vi "CMC_Homework_02.vi"() -> ()   [LabVIEW 2013]
doc: "Simulates the hardware controls for a manufacturing machine\nCreated in part with the collaboration of Sarah Bailey & Alex Offredi"
panel:
  in  "Max Tank Pressure":dbl(knob)=875.0 scale=0.0..10.0
  in  "Max Tank Temp":dbl(knob)=550.0 scale=0.0..10.0
  in  "Max Ps":dbl(knob)=700.0 scale=0.0..10.0
  in  "Max Ts":dbl(knob)=230.0 scale=0.0..10.0
  in  "Tank Pressure":dbl(knob) step=1.0 scale=0.0..1000.0
  in  "Tank Temp":dbl(knob) step=1.0 scale=0.0..1000.0
  out "Status":string
  in  "stop":bool
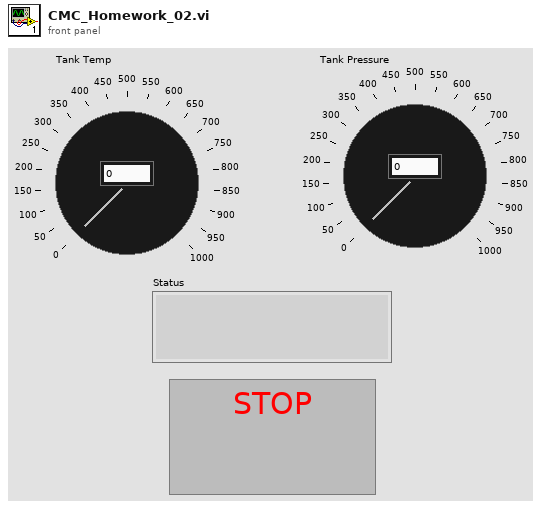
[diagram p1: front panel]
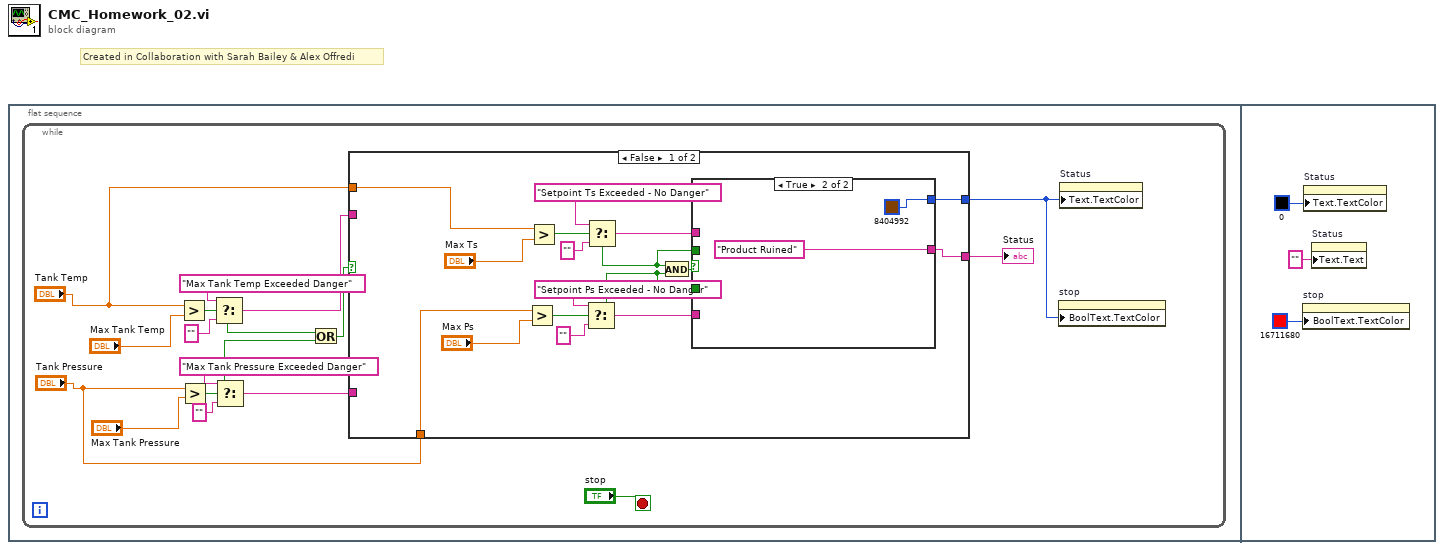
[diagram p0: block diagram]
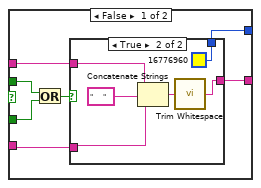
[diagram p2: hidden frame]
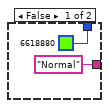
[diagram p3: hidden frame]
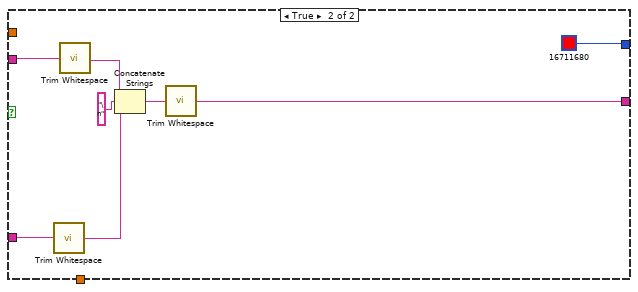
[diagram p4: hidden frame]
diagram:
  # "Created in Collaboration with Sarah Bailey & Alex Offredi"
  n1 = flat-sequence {
    frame #0 {
      n2 = while {
        stop <- "stop" stop-if-true
        n3 = Greater?(x="Tank Temp", y="Max Tank Temp") -> (0:w10:bool)
        n4 = Greater?(x="Tank Pressure", y="Max Tank Pressure") -> (0:w9:bool)
        n5 = Select(t="Max Tank Temp Exceeded Danger", s=w10, f="") -> (s? t:f=w7:string)
        n6 = Select(t="Max Tank Pressure Exceeded Danger", s=w9, f="") -> (s? t:f=w6:string)
        n7 = Or(x=w10, y=w9) -> (x .or. y?=w8:bool)
        n8 = case shown="False" w8 {
          tunnel: w7 -> [_ w53]
          tunnel: w6 -> [_ w52]
          tunnel: [w20 w49] -> w5
          tunnel: "Tank Temp" -> [w19 _]
          tunnel: "Tank Pressure" -> [w18 _]
          tunnel: [w17 u32 16711680] -> w1
          frame False {
            n9 = Greater?(x=w18, y="Max Ps") -> (0:w21:bool)
            n10 = Greater?(x=w19, y="Max Ts") -> (0:w22:bool)
            n11 = Select(t="Setpoint Ps Exceeded - No Danger", s=w21, f="") -> (s? t:f=w23:string)
            n12 = Select(t="Setpoint Ts Exceeded - No Danger", s=w22, f="") -> (s? t:f=w24:string)
            n13 = And(x=w22, y=w21) -> (x .and. y?=w25:bool)
            n14 = case shown="True" w25 {
              tunnel: w24 -> [w35 _]
              tunnel: w23 -> [w34 _]
              tunnel: [w33 "Product Ruined"] -> w20
              tunnel: w22 -> [w37 _]
              tunnel: w21 -> [w36 _]
              tunnel: [w32 u32 8404992] -> w17
              frame False {
                n15 = Or(x=w37, y=w36) -> (x .or. y?=w38:bool)
                n16 = case shown="True" w38 {
                  tunnel: w35 -> [_ w46]
                  tunnel: w34 -> [_ w45]
                  tunnel: ["Normal" w42] -> w33
                  tunnel: [u32 6618880 u32 16776960] -> w32
                  frame False {
                  }
                  frame True {
                    n17 = Concatenate Strings(w46, "     ", w45) -> (w43:string)
                    n18 = call <vilib>:"Trim Whitespace.vi"("string"=w43) -> ("trimmed string"=w42:string)  [unwired: 1 in]
                  }
                }
              }
              frame True {
              }
            }
          }
          frame True {
            n19 = call <vilib>:"Trim Whitespace.vi"("string"=w52) -> ("trimmed string"=w51:string)  [unwired: 1 in]
            n20 = call <vilib>:"Trim Whitespace.vi"("string"=w53) -> ("trimmed string"=w54:string)  [unwired: 1 in]
            n21 = Concatenate Strings(w54, "\n" ("string"), w51) -> (w50:string)
            n22 = call <vilib>:"Trim Whitespace.vi"("string"=w50) -> ("trimmed string"=w49:string)  [unwired: 1 in]
          }
        }
        "Status" <- w5
        n23 = property on="stop" class="Bool"("BoolText.TextColor"=w1) -> ()  [unwired: 2 in, 2 out]
        n24 = property on="Status" class="Str"("Text.TextColor"=w1) -> ()  [unwired: 2 in, 2 out]
      }
    }
    frame #1 {
      n25 = property on="stop" class="Bool"("BoolText.TextColor"=u32 16711680) -> ()  [unwired: 2 in, 2 out]
      n26 = property on="Status" class="Str"("Text.TextColor"=u32 0) -> ()  [unwired: 2 in, 2 out]
      n27 = property on="Status" class="Str"("Text.Text"="") -> ()  [unwired: 2 in, 2 out]
    }
  }
